vi "TCP Query Ophir.vi"(11 "error in":errorcluster) -> (4 "Energy":dbl, 6 "timestring":string, 8 "Status":string, 10 "Range":i32, 15 "error out":errorcluster)   [LabVIEW 2013]
panel:
  out "array":string[](array[string])
  out "data out":string
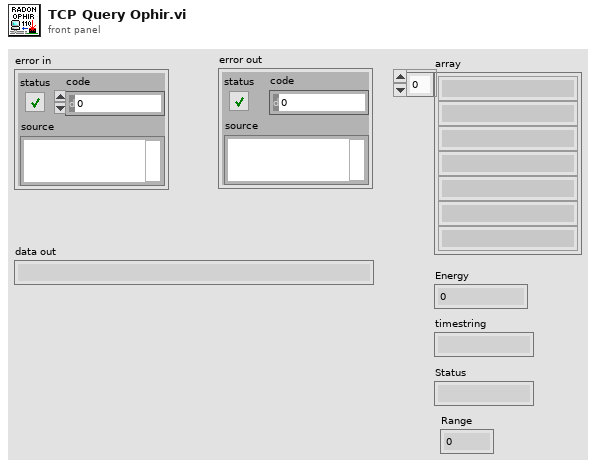
[diagram p1: front panel]
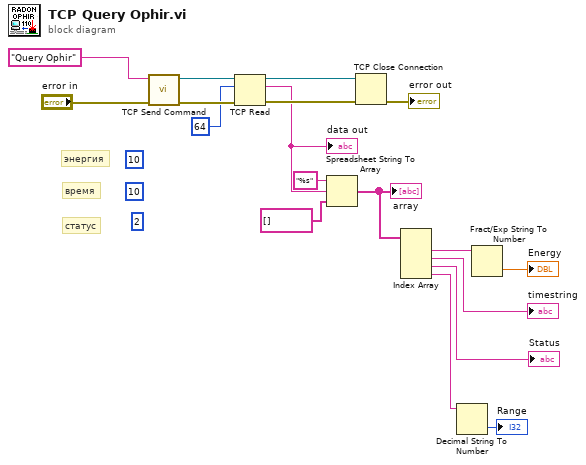
[diagram p0: block diagram]
diagram:
  (unwired) 2 ("bytes to read")
  (unwired) 10 ("bytes to read")
  (unwired) 10 ("bytes to read")
  # "статус"
  # "время"
  # "энергия"
  n1 = call "TCP Send Command.vi"("error in"="error in", "Command"="Query Ophir") -> ("error out"=w16:errorcluster, "connection ID out"=w15:refnum<k5>)  [unwired: 8 in]
  n2 = TCP Read(connection ID=w15, bytes to read=64, error in (no error)=w16) -> (connection ID out=w12:refnum<k5>, data out=w10:string, error out=w13:errorcluster)  [unwired: 2 in]
  "data out" <- w10
  n3 = Spreadsheet String To Array(format string="%s", spreadsheet string=w10, array type (2D Dbl)=string[] []) -> (array=w7:string[])  [unwired: 1 in]
  "array" <- w7
  n4 = TCP Close Connection(connection ID=w12, error in (no error)=w13) -> (error out=→"error out":errorcluster)  [unwired: 1 in, 1 out]
  n5 = Index Array(array=w7) -> (element #1=w6:string, element #2=→"timestring":string, element #3=→"Status":string, element #4=w2:string)  [unwired: 4 in]
  n6 = Decimal String To Number(string=w2) -> (number=→"Range":i32)  [unwired: 2 in, 1 out]
  n7 = Fract/Exp String To Number(string=w6) -> (number=→"Energy":dbl)  [unwired: 3 in, 1 out]
